vi "Construct sqlite3.vi"(8 "error in (no error)":errorcluster, 10 "DatabaseFilePath":path) -> (0 "error out":errorcluster, 3 "sqlite3 out":refnum<class "sqlite3.lvclass">)   [LabVIEW 2020, in "sqlite3.lvlib" / "sqlite3.lvclass"]
uses:
  sqlite3.lvclass
  sqlite3.lvclass/sqlite3.ctl
  <vilib>/Utility/error.llb/Error Cluster From Error Code.vi
  <vilib>/ErrorRing/Error Ring.xnode
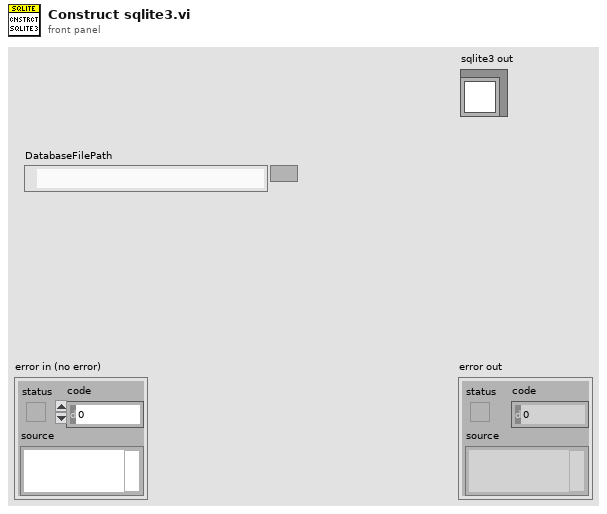
[diagram p1: front panel]
types:
  T1 = enum16{"open", "replace", "create", "open or create", "replace or create", "replace or create with confirmation"}
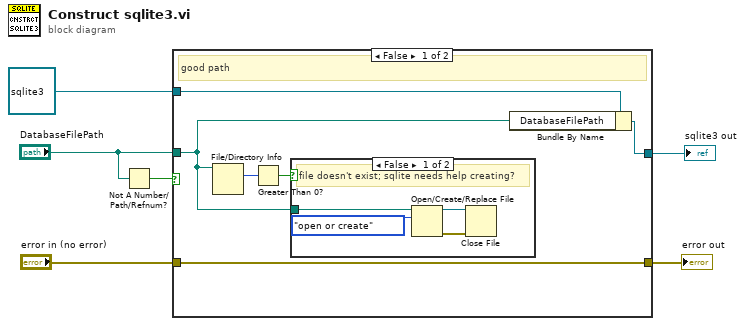
[diagram p0: block diagram]
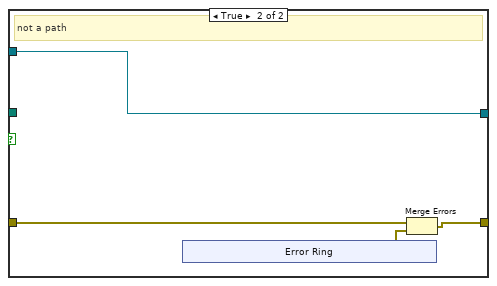
[diagram p3: hidden frame]
diagram:
  n1 = Not A Number/Path/Refnum?(number/path/refnum="DatabaseFilePath") -> (NaN/Path/Refnum?=w6:bool)
  n2 = case shown="False" w6 {
    tunnel: "error in (no error)" -> [w10 w20]
    tunnel: [w10 w18] -> w4
    tunnel: refnum<class "sqlite3.lvclass"> refnum ("sqlite3 out") -> [w12 w19]
    tunnel: "DatabaseFilePath" -> [w7 _]
    tunnel: [w11 w19] -> w1
    frame False {
      # "good path"
      n3 = File/Directory Info(path=w7) -> (size=w9:i64)  [unwired: 1 in, 6 out]
      n4 = Greater Than 0?(x=w9) -> (x > 0?=w8:bool)
      n5 = case shown="False" w8 {
        tunnel: w7 -> [w16 _]
        frame False {
          # "file doesn't exist; sqlite needs help creating?"
          n6 = Open/Create/Replace File(file path (use dialog)=w16, operation (0:open)=T1."open or create") -> (refnum out=w14:refnum<file>, error out=w13:errorcluster)  [unwired: 4 in, 1 out]
          n7 = Close File(refnum=w14, error in=w13) -> ()  [unwired: 2 out]
        }
        frame True {
        }
      }
      n8 = Bundle By Name(cluster=w12, "DatabaseFilePath"=w7) -> (w11:refnum<class "sqlite3.lvclass">)
    }
    frame True {
      # "not a path"
      n9 = xnode "Error Ring"() -> ("error out"=w17:errorcluster)
      n10 = Merge Errors(w20, w17) -> (w18:errorcluster)
    }
  }
  "error out" <- w4
  "sqlite3 out" <- w1
